vi "Write Cursor.vi"(8 "error in (no error)":errorcluster, 9 "Cursor On":bool, 10 "Session In":refnum<class "Session.lvclass">, 11 "Char LCD I in":refnum<class "Char LCD.lvclass">) -> (0 "error out":errorcluster, 2 "Session Out":refnum<class "Session.lvclass">, 3 "Char LCD I out":refnum<class "Char LCD.lvclass">)   [LabVIEW 2020, in "CTI-Peripheral.lvlib" / "Char LCD.lvclass"]
uses:
  Char LCD.lvclass
  CTI/Session/Session.lvclass
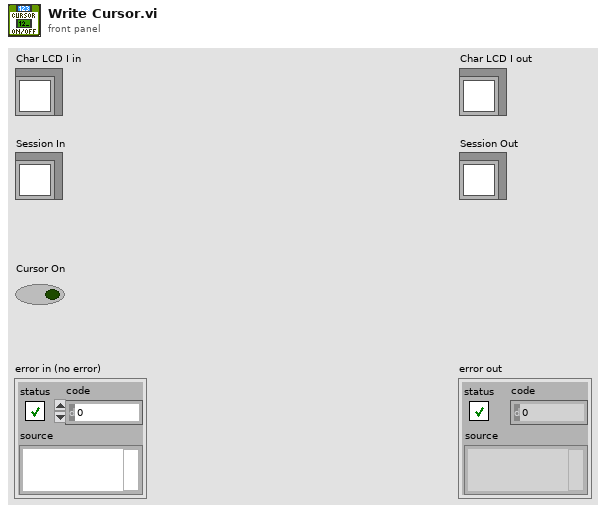
[diagram p1: front panel]
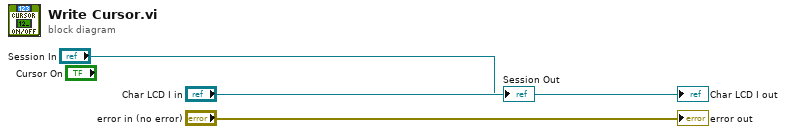
[diagram p0: block diagram]
diagram:
  "error out" <- "error in (no error)"
  "Char LCD I out" <- "Char LCD I in"
  "Session Out" <- "Session In"
